vi "Set Gripper.vi"(8 "error in (no error)":errorcluster, 10 "KUKA youBot gripper":refnum<class "NI_Robotics_KUKA youBot Gripper.lvclass">, 11 "KUKA youBot arm in":refnum<class "NI_Robotics_KUKA youBot Arm.lvclass">) -> (0 "error out":errorcluster, 3 "KUKA youBot arm out":refnum<class "NI_Robotics_KUKA youBot Arm.lvclass">)   [LabVIEW 2017, in "NI_Robotics_KUKA youBot Host.lvlib" / "NI_Robotics_KUKA youBot Arm.lvclass"]
uses:
  <vilib>/robotics/KUKA youBot/Basic Device/Arm/NI_Robotics_KUKA youBot Arm.lvclass
  <vilib>/robotics/KUKA youBot/Basic Device/Gripper/NI_Robotics_KUKA youBot Gripper.lvclass
  <vilib>/robotics/KUKA youBot/Basic Device/Arm/NI_Robotics_KUKA youBot Arm.lvclass/NI_Robotics_KUKA youBot Arm.ctl
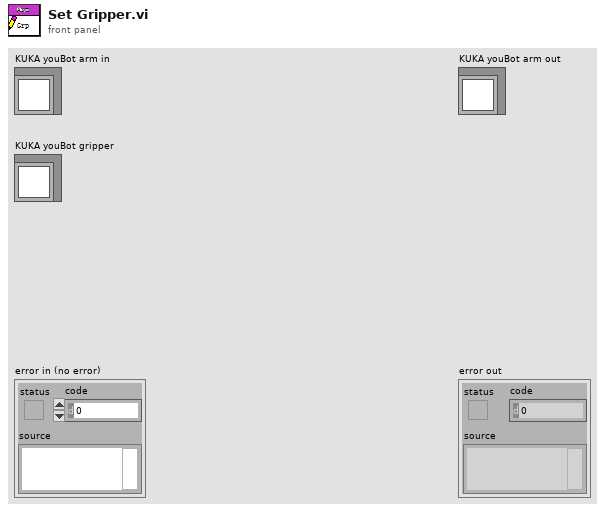
[diagram p1: front panel]
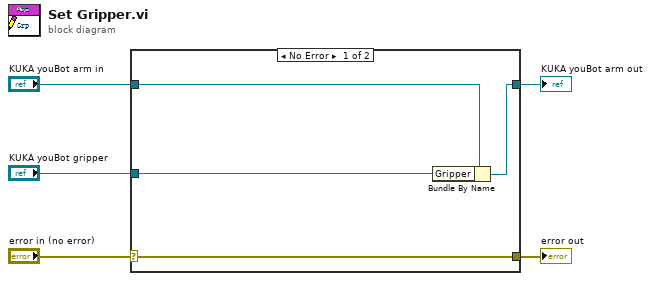
[diagram p0: block diagram]
diagram:
  n1 = case shown="No Error" "error in (no error)" {
    selector: "error in (no error)" -> [w9 w10]
    tunnel: [w9 w10] -> w4
    tunnel: [w7 w11] -> w2
    tunnel: "KUKA youBot arm in" -> [w8 w11]
    tunnel: "KUKA youBot gripper" -> [w6 _]
    frame No Error {
      n2 = Bundle By Name(cluster=w8, "Gripper"=w6) -> (w7:refnum<class "NI_Robotics_KUKA youBot Arm.lvclass">)
    }
    frame Error {
    }
  }
  "error out" <- w4
  "KUKA youBot arm out" <- w2
